vi "Start New File.vi"(8 "error in (no error)":errorcluster, 11 "Log in":refnum<class "Log.lvclass">) -> (0 "error out":errorcluster, 3 "Log out":refnum<class "Log.lvclass">)   [LabVIEW 2020, in "Log.lvclass"]
doc: "Derive the next filename in the incrementing sequence and store in Current Path."
uses:
  Log.lvclass
  Log.lvclass/Log.ctl
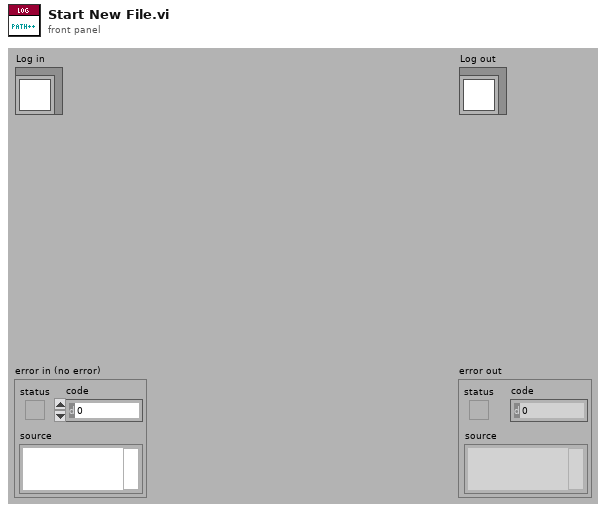
[diagram p1: front panel]
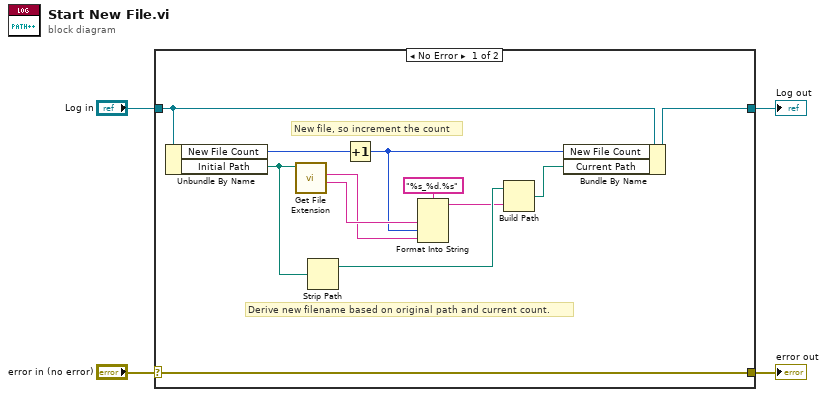
[diagram p0: block diagram]
diagram:
  n1 = case shown="No Error" "error in (no error)" {
    selector: "error in (no error)" -> [w9 w18]
    tunnel: [w9 w18] -> w3
    tunnel: [w6 w17] -> w1
    tunnel: "Log in" -> [w7 w17]
    frame No Error {
      # "New file, so increment the count"
      # "Derive new filename based on original path and current count."
      n2 = Unbundle By Name(w7) -> ("New File Count"=w16:i32, "Initial Path"=w12:path)
      n3 = call <vilib>:"Get File Extension.vi"("file"=w12) -> ("filename without extension"=w14:string, "lowercase file extension"=w13:string)  [unwired: 1 in, 8 out]
      n4 = Strip Path(path=w12) -> (stripped path=w11:path)  [unwired: 1 out]
      n5 = Increment(x=w16) -> (x+1=w5:i32)
      n6 = Format Into String(format string="%s_%d.%s", w14, w5, w13) -> (resulting string=w10:string)  [unwired: 2 in, 1 out]
      n7 = Build Path(base path=w11, name or relative path=w10) -> (appended path=w8:path)
      n8 = Bundle By Name(cluster=w7, "New File Count"=w5, "Current Path"=w8) -> (w6:refnum<class "Log.lvclass">)
    }
    frame Error {
    }
  }
  "error out" <- w3
  "Log out" <- w1
